vi "U16 to 2 byte array.vi"(0 "Numeric":u16) -> (1 "2byte U16":u8[](array[numeric]), 2 "Num of bytes":u8)   [LabVIEW 2017]
doc: "Converts an unsigned 16 bit integer (U16) to an array of 2 bytes.\nElement 0 = MSB\nElement 1 = LSB"
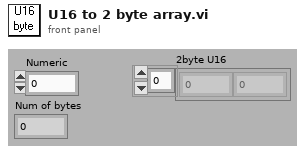
[diagram p1: front panel]
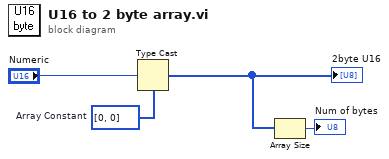
[diagram p0: block diagram]
diagram:
  w4 = u8[] [0, 0]  # Array Constant
  n1 = Type Cast(type=w4, x="Numeric") -> (*(type *) &x=w1:u8[])
  "2byte U16" <- w1
  n2 = Array Size(array=w1) -> (size(s)=→"Num of bytes":i32)
